vi "Circle.vi"(10 "Min/Max Voltage":dbl format="%#_13g") -> (0 "Rate":dbl=12800.0, 2 "Scanners trajectories":dbl[][](graph)=[[0.0, 0.003925413946193441, 0.007841371226364848, 0.01173843795642894, 0.015607225761290262, 0.019438414392261114, 0.02322277418035699, 0.02695118827137761, 0.030614674589207184, 0.03420440747442258, 0.03771173894607982, 0.04112821953545775, 0.04444561864156819, 0.04765594435939468, 0.050751462733091654, 0.05372471638776148, 0.05656854249492382, 0.05927609002839673, 0.06184083626901897, 0.0642566025184516, 0.06651756898420363, 0.06861828880002177, 0.07055370114786842, 0.07231914344987547, 0.07391036260090296, 0.07532352521464167, 0.07655522685857673, 0.07760250025556352, 0.07846282243225845, 0.07913412079718248, 0.07961477813377577, 0.07990363649641379, 0.08, 0.07990363649641379, 0.07961477813377575, 0.07913412079718248, 0.07846282243225844, 0.07760250025556352, 0.07655522685857671, 0.07532352521464167, 0.07391036260090295, 0.07231914344987547, 0.07055370114786841, 0.06861828880002177, 0.06651756898420362, 0.0642566025184516, 0.061840836269018956, 0.05927609002839673, 0.0565685424949238, 0.05372471638776148, 0.05075146273309164, 0.04765594435939468, 0.04444561864156818, 0.04112821953545775, 0.03771173894607981, 0.03420440747442258, 0.030614674589207184, 0.026951188271377612, 0.023222774180356995, 0.01943841439226112, 0.01560722576129027, 0.011738437956428949, 0.007841371226364857, 0.003925413946193449, 1.0408340855860843e-17, -0.0039254139461934335, -0.007841371226364836, -0.011738437956428933, -0.015607225761290248, -0.019438414392261107, -0.023222774180356974, -0.026951188271377602, -0.030614674589207164, -0.03420440747442256, -0.03771173894607979, -0.041128219535457734, -0.04444561864156816, -0.047655944359394665, -0.05075146273309162, -0.05372471638776147, -0.05656854249492378, -0.05927609002839672, -0.061840836269018935, -0.06425660251845158, -0.06651756898420359, -0.06861828880002176, -0.07055370114786838, -0.07231914344987546, -0.07391036260090292, -0.07532352521464165, -0.07655522685857669, -0.0776025002555635, -0.07846282243225841, -0.07913412079718246, -0.07961477813377572, -0.07990363649641377, -0.07999999999999997, -0.07990363649641377, -0.07961477813377572, -0.07913412079718246, -0.07846282243225841, -0.0776025002555635, -0.07655522685857669, -0.07532352521464165, -0.07391036260090292, -0.07231914344987546, -0.07055370114786838, -0.06861828880002176, -0.06651756898420359, -0.06425660251845158, -0.061840836269018935, -0.05927609002839672, -0.05656854249492378, -0.05372471638776147, -0.050751462733091626, -0.047655944359394665, -0.044445618641568166, -0.04112821953545774, -0.037711738946079806, -0.03420440747442257, -0.030614674589207178, -0.02695118827137761, -0.023222774180356988, -0.019438414392261117, -0.015607225761290264, -0.011738437956428947, -0.007841371226364855, -0.003925413946193451], [0.08, 0.0799036364964138, 0.07961477813377575, 0.07913412079718249, 0.07846282243225844, 0.07760250025556353, 0.07655522685857671, 0.07532352521464168, 0.07391036260090295, 0.07231914344987549, 0.07055370114786841, 0.06861828880002178, 0.06651756898420362, 0.06425660251845161, 0.061840836269018956, 0.05927609002839675, 0.0565685424949238, 0.053724716387761495, 0.05075146273309164, 0.04765594435939469, 0.04444561864156818, 0.04112821953545776, 0.03771173894607981, 0.03420440747442259, 0.030614674589207184, 0.026951188271377626, 0.02322277418035699, 0.019438414392261134, 0.015607225761290262, 0.011738437956428963, 0.00784137122636485, 0.003925413946193463, 1.734723475976807e-18, -0.00392541394619342, -0.007841371226364847, -0.01173843795642892, -0.015607225761290259, -0.019438414392261093, -0.023222774180356988, -0.026951188271377588, -0.03061467458920718, -0.03420440747442255, -0.03771173894607981, -0.04112821953545772, -0.04444561864156818, -0.04765594435939465, -0.05075146273309164, -0.053724716387761454, -0.0565685424949238, -0.059276090028396705, -0.061840836269018956, -0.06425660251845157, -0.06651756898420362, -0.06861828880002174, -0.07055370114786841, -0.07231914344987544, -0.07391036260090295, -0.07532352521464164, -0.07655522685857671, -0.07760250025556349, -0.07846282243225844, -0.07913412079718245, -0.07961477813377575, -0.07990363649641376, -0.08, -0.07990363649641376, -0.07961477813377575, -0.07913412079718245, -0.07846282243225844, -0.07760250025556349, -0.07655522685857671, -0.07532352521464164, -0.07391036260090295, -0.07231914344987544, -0.07055370114786841, -0.06861828880002174, -0.06651756898420362, -0.06425660251845157, -0.061840836269018956, -0.059276090028396705, -0.0565685424949238, -0.053724716387761454, -0.05075146273309164, -0.04765594435939465, -0.04444561864156818, -0.04112821953545773, -0.03771173894607981, -0.034204407474422556, -0.030614674589207184, -0.026951188271377595, -0.023222774180356995, -0.019438414392261103, -0.01560722576129027, -0.011738437956428933, -0.007841371226364857, -0.003925413946193437, -1.0408340855860843e-17, 0.003925413946193442, 0.007841371226364836, 0.011738437956428939, 0.015607225761290248, 0.019438414392261107, 0.023222774180356974, 0.0269511882713776, 0.030614674589207164, 0.03420440747442256, 0.03771173894607979, 0.041128219535457734, 0.04444561864156816, 0.04765594435939466, 0.05075146273309162, 0.05372471638776146, 0.05656854249492378, 0.05927609002839671, 0.061840836269018935, 0.06425660251845157, 0.06651756898420359, 0.06861828880002174, 0.07055370114786838, 0.07231914344987544, 0.07391036260090292, 0.07532352521464164, 0.07655522685857669, 0.07760250025556349, 0.07846282243225841, 0.07913412079718245, 0.07961477813377572, 0.07990363649641376]], 3 "XY Graph":cluster{"sine wave":dbl[], "sine wave":dbl[]}(graph)={"sine wave"=[0.0, 0.003925413946193441, 0.007841371226364848, 0.01173843795642894, 0.015607225761290262, 0.019438414392261114, 0.02322277418035699, 0.02695118827137761, 0.030614674589207184, 0.03420440747442258, 0.03771173894607982, 0.04112821953545775, 0.04444561864156819, 0.04765594435939468, 0.050751462733091654, 0.05372471638776148, 0.05656854249492382, 0.05927609002839673, 0.06184083626901897, 0.0642566025184516, 0.06651756898420363, 0.06861828880002177, 0.07055370114786842, 0.07231914344987547, 0.07391036260090296, 0.07532352521464167, 0.07655522685857673, 0.07760250025556352, 0.07846282243225845, 0.07913412079718248, 0.07961477813377577, 0.07990363649641379, 0.08, 0.07990363649641379, 0.07961477813377575, 0.07913412079718248, 0.07846282243225844, 0.07760250025556352, 0.07655522685857671, 0.07532352521464167, 0.07391036260090295, 0.07231914344987547, 0.07055370114786841, 0.06861828880002177, 0.06651756898420362, 0.0642566025184516, 0.061840836269018956, 0.05927609002839673, 0.0565685424949238, 0.05372471638776148, 0.05075146273309164, 0.04765594435939468, 0.04444561864156818, 0.04112821953545775, 0.03771173894607981, 0.03420440747442258, 0.030614674589207184, 0.026951188271377612, 0.023222774180356995, 0.01943841439226112, 0.01560722576129027, 0.011738437956428949, 0.007841371226364857, 0.003925413946193449, 1.0408340855860843e-17, -0.0039254139461934335, -0.007841371226364836, -0.011738437956428933, -0.015607225761290248, -0.019438414392261107, -0.023222774180356974, -0.026951188271377602, -0.030614674589207164, -0.03420440747442256, -0.03771173894607979, -0.041128219535457734, -0.04444561864156816, -0.047655944359394665, -0.05075146273309162, -0.05372471638776147, -0.05656854249492378, -0.05927609002839672, -0.061840836269018935, -0.06425660251845158, -0.06651756898420359, -0.06861828880002176, -0.07055370114786838, -0.07231914344987546, -0.07391036260090292, -0.07532352521464165, -0.07655522685857669, -0.0776025002555635, -0.07846282243225841, -0.07913412079718246, -0.07961477813377572, -0.07990363649641377, -0.07999999999999997, -0.07990363649641377, -0.07961477813377572, -0.07913412079718246, -0.07846282243225841, -0.0776025002555635, -0.07655522685857669, -0.07532352521464165, -0.07391036260090292, -0.07231914344987546, -0.07055370114786838, -0.06861828880002176, -0.06651756898420359, -0.06425660251845158, -0.061840836269018935, -0.05927609002839672, -0.05656854249492378, -0.05372471638776147, -0.050751462733091626, -0.047655944359394665, -0.044445618641568166, -0.04112821953545774, -0.037711738946079806, -0.03420440747442257, -0.030614674589207178, -0.02695118827137761, -0.023222774180356988, -0.019438414392261117, -0.015607225761290264, -0.011738437956428947, -0.007841371226364855, -0.003925413946193451], "sine wave"=[0.08, 0.0799036364964138, 0.07961477813377575, 0.07913412079718249, 0.07846282243225844, 0.07760250025556353, 0.07655522685857671, 0.07532352521464168, 0.07391036260090295, 0.07231914344987549, 0.07055370114786841, 0.06861828880002178, 0.06651756898420362, 0.06425660251845161, 0.061840836269018956, 0.05927609002839675, 0.0565685424949238, 0.053724716387761495, 0.05075146273309164, 0.04765594435939469, 0.04444561864156818, 0.04112821953545776, 0.03771173894607981, 0.03420440747442259, 0.030614674589207184, 0.026951188271377626, 0.02322277418035699, 0.019438414392261134, 0.015607225761290262, 0.011738437956428963, 0.00784137122636485, 0.003925413946193463, 1.734723475976807e-18, -0.00392541394619342, -0.007841371226364847, -0.01173843795642892, -0.015607225761290259, -0.019438414392261093, -0.023222774180356988, -0.026951188271377588, -0.03061467458920718, -0.03420440747442255, -0.03771173894607981, -0.04112821953545772, -0.04444561864156818, -0.04765594435939465, -0.05075146273309164, -0.053724716387761454, -0.0565685424949238, -0.059276090028396705, -0.061840836269018956, -0.06425660251845157, -0.06651756898420362, -0.06861828880002174, -0.07055370114786841, -0.07231914344987544, -0.07391036260090295, -0.07532352521464164, -0.07655522685857671, -0.07760250025556349, -0.07846282243225844, -0.07913412079718245, -0.07961477813377575, -0.07990363649641376, -0.08, -0.07990363649641376, -0.07961477813377575, -0.07913412079718245, -0.07846282243225844, -0.07760250025556349, -0.07655522685857671, -0.07532352521464164, -0.07391036260090295, -0.07231914344987544, -0.07055370114786841, -0.06861828880002174, -0.06651756898420362, -0.06425660251845157, -0.061840836269018956, -0.059276090028396705, -0.0565685424949238, -0.053724716387761454, -0.05075146273309164, -0.04765594435939465, -0.04444561864156818, -0.04112821953545773, -0.03771173894607981, -0.034204407474422556, -0.030614674589207184, -0.026951188271377595, -0.023222774180356995, -0.019438414392261103, -0.01560722576129027, -0.011738437956428933, -0.007841371226364857, -0.003925413946193437, -1.0408340855860843e-17, 0.003925413946193442, 0.007841371226364836, 0.011738437956428939, 0.015607225761290248, 0.019438414392261107, 0.023222774180356974, 0.0269511882713776, 0.030614674589207164, 0.03420440747442256, 0.03771173894607979, 0.041128219535457734, 0.04444561864156816, 0.04765594435939466, 0.05075146273309162, 0.05372471638776146, 0.05656854249492378, 0.05927609002839671, 0.061840836269018935, 0.06425660251845157, 0.06651756898420359, 0.06861828880002174, 0.07055370114786838, 0.07231914344987544, 0.07391036260090292, 0.07532352521464164, 0.07655522685857669, 0.07760250025556349, 0.07846282243225841, 0.07913412079718245, 0.07961477813377572, 0.07990363649641376]})   [LabVIEW 2021]
doc: "This VI enables to display the Circle optotype.\n\nInput:\n(1) Min/Max Voltage - the absolute value of the Voltage. Due to this parameter, the size of the optotype can be changed. Voltage about 10V is not allowed.\n\nOutputs: \n(1) XY Graph - the optotype data, to display the pattern.\n(2) Scanners trajectories - the XY data for the Scanners.\n(3) Rate - the rate parameter equal to 12800."
uses:
  <vilib>/Utility/error.llb/DialogType.ctl
  <vilib>/Analysis/NI_AALBase.lvlib
panel:
  out "Y-scanner trajectory":dbl[](array[numeric])
  out "X-scanner trajectory":dbl[](array[numeric])
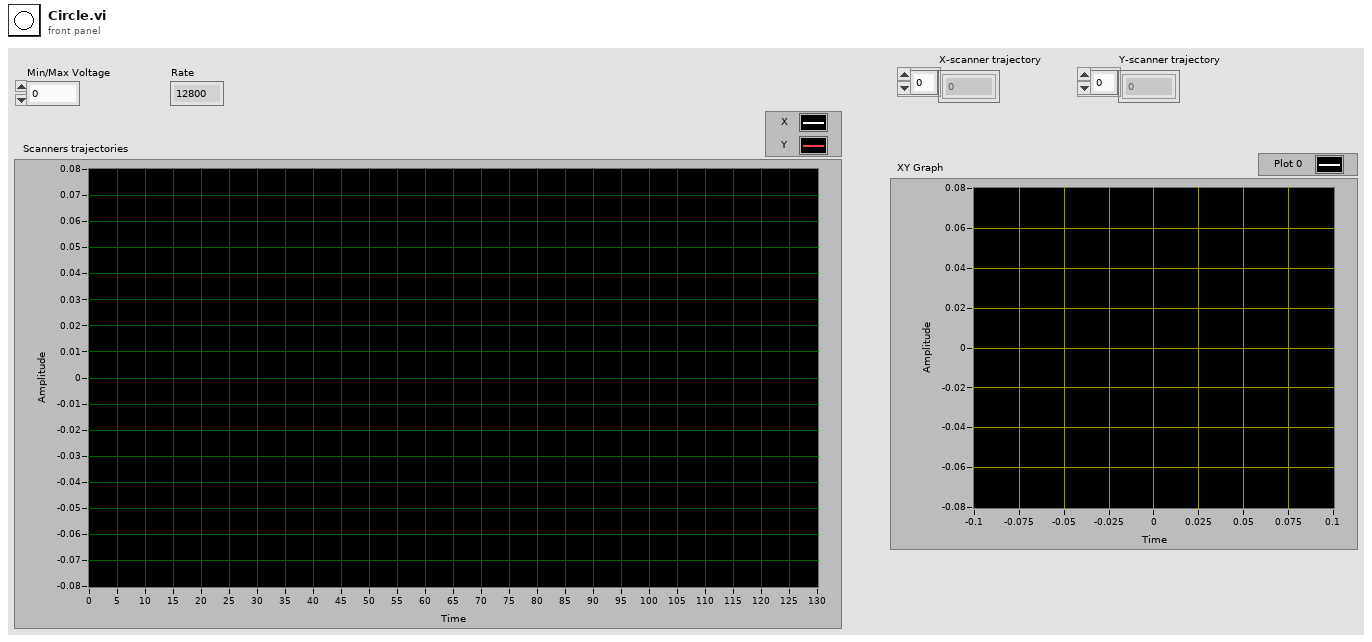
[diagram p1: front panel]
types:
  T1 = typedef "DialogType.ctl" = u16
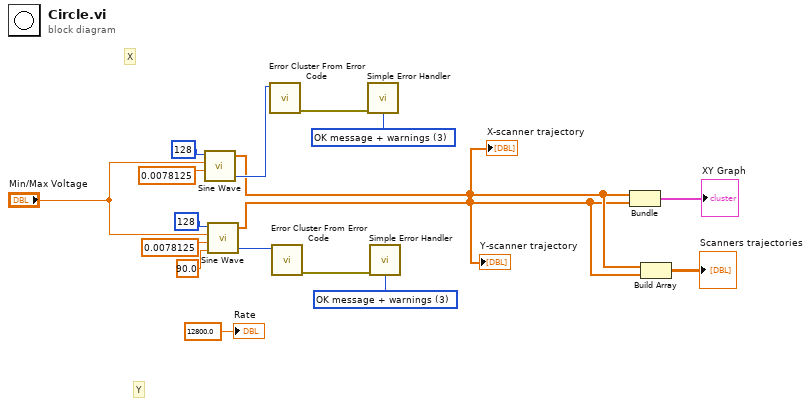
[diagram p0: block diagram]
diagram:
  w9 = T1 3 items=["no dialog", "OK message", "continue or stop message", "OK message + warnings", "continue/stop + warnings"] ("type of dialog (OK msg:1)")
  w11 = T1 3 items=["no dialog", "OK message", "continue or stop message", "OK message + warnings", "continue/stop + warnings"] ("type of dialog (OK msg:1)")
  # "Y"
  # "X"
  n1 = call <vilib>:"Sine Wave.vi"("samples"=128, "amplitude"="Min/Max Voltage", "frequency"=0.0078125) -> ("sine wave"=w5:dbl[], "error"=w7:i32)  [unwired: 2 in, 1 out]
  "X-scanner trajectory" <- w5
  n2 = call <vilib>:"Sine Wave.vi"("samples"=128, "amplitude"="Min/Max Voltage", "frequency"=0.0078125, "phase in"=90.0) -> ("sine wave"=w4:dbl[], "error"=w12:i32)  [unwired: 1 in, 1 out]
  "Y-scanner trajectory" <- w4
  n3 = call <vilib>:"Error Cluster From Error Code.vi"("error code (0)"=w7) -> ("error out"=w8:errorcluster)  [unwired: 8 in]
  n4 = call <vilib>:"Error Cluster From Error Code.vi"("error code (0)"=w12) -> ("error out"=w10:errorcluster)  [unwired: 8 in]
  n5 = call <vilib>:"Simple Error Handler.vi"("type of dialog (OK msg:1)"=w9, "error in (no error)"=w8) -> ()  [unwired: 3 in, 5 out]
  n6 = call <vilib>:"Simple Error Handler.vi"("type of dialog (OK msg:1)"=w11, "error in (no error)"=w10) -> ()  [unwired: 3 in, 5 out]
  n7 = Bundle("sine wave"=w5, "sine wave"=w4) -> (→"XY Graph":cluster{"sine wave":dbl[], "sine wave":dbl[]})  [unwired: 1 in]
  n8 = Build Array(w5, w4) -> (→"Scanners trajectories":dbl[][])
  "Rate" <- 12800.0
